vi "FT10_Fornax Read.vi"(8 "error in (no error)":errorcluster, 10 "Timeout":dbl, 11 "TCP Network Connection in":refnum<k5>) -> (0 "error out":errorcluster, 2 "JSON Message":string[](array[string]), 3 "TCP Network Connection out":refnum<k5>)   [LabVIEW 2015]
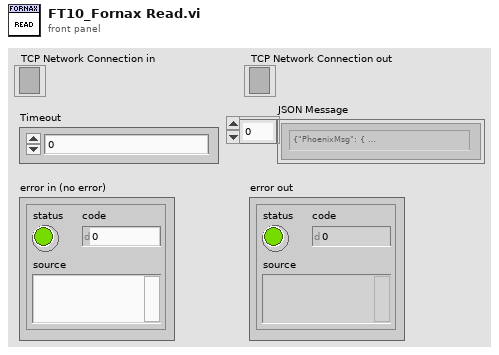
[diagram p1: front panel]
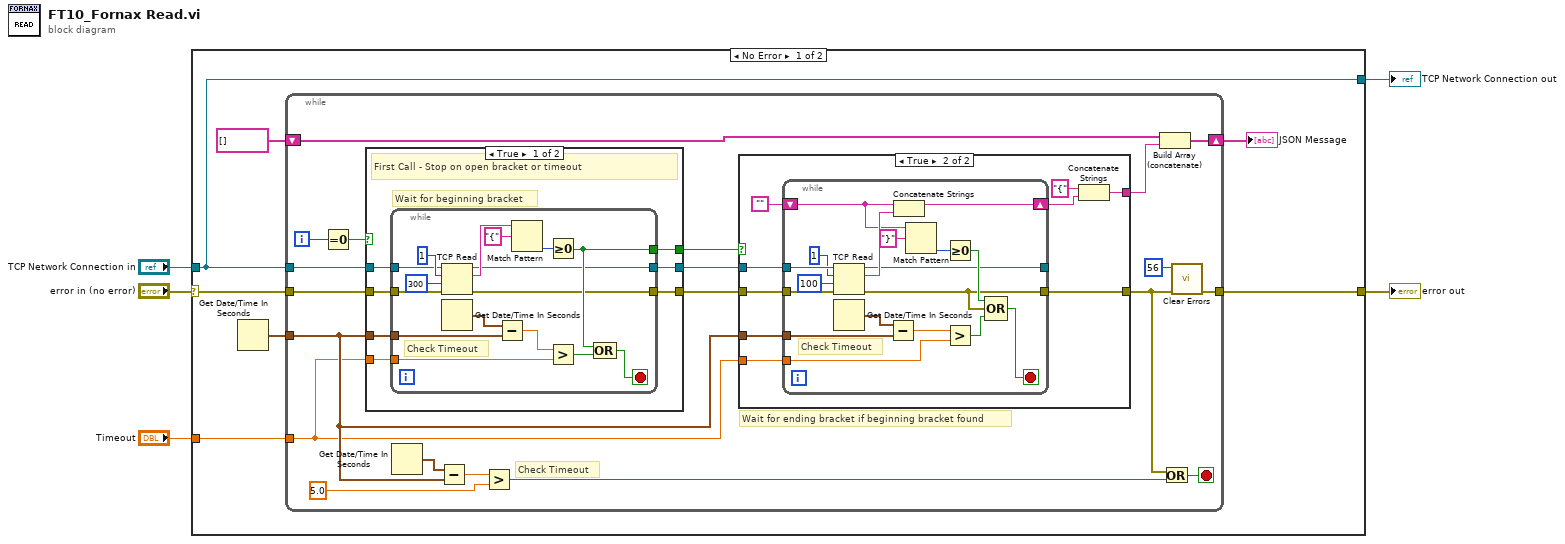
[diagram p0: block diagram]
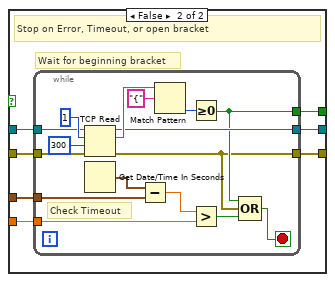
[diagram p2: hidden frame]
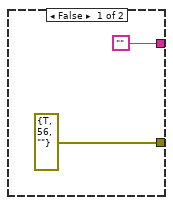
[diagram p3: hidden frame]
diagram:
  n1 = case shown="No Error" "error in (no error)" {
    selector: "error in (no error)" -> [w12 w109]
    tunnel: [w10 w109] -> w2
    tunnel: "TCP Network Connection in" -> [w9 w108]
    tunnel: [w9 w108] -> w4
    tunnel: "Timeout" -> [w8 _]
    frame No Error {
      n2 = Get Date/Time In Seconds() -> (seconds since 1Jan1904=w11:timestamp)
      n3 = while {
        tunnel: w12 -> [w22]
        tunnel: w11 -> [w25]
        tunnel: [w24] -> w10
        tunnel: w8 -> [w20]
        tunnel: w9 -> [w31]
        shift-right: [w17] -> w7
        shift-left: string[] [] ("appended array") -> [w16]
        i -> [w15]
        stop <- w27 stop-if-true
        # "Check Timeout"
        # "Wait for ending bracket if beginning bracket found"
        n4 = Equal To 0?(x=w15) -> (x = 0?=w14:bool)
        n5 = case shown="True" w14 {
          tunnel: [w39 w62] -> w32
          tunnel: w31 -> [w38 w61]
          tunnel: [w37 w60] -> w30
          tunnel: w25 -> [w36 w59]
          tunnel: w22 -> [w35 w58]
          tunnel: w20 -> [w34 w57]
          tunnel: [w33 w56] -> w19
          frame True {
            # "Wait for beginning bracket"
            # "First Call - Stop on open bracket or timeout"
            n6 = while {
              tunnel: w35 -> [w53]
              tunnel: w38 -> [w52]
              tunnel: [w44] -> w39
              tunnel: w36 -> [w48]
              tunnel: [w45] -> w37
              tunnel: w34 -> [w41]
              tunnel: [w40] -> w33
              stop <- w43 stop-if-true
              # "Check Timeout"
              n7 = TCP Read(connection ID=w52, bytes to read=1, error in (no error)=w53, 9:300) -> (connection ID out=w40:refnum<k5>, data out=w47:string, error out=w44:errorcluster)  [unwired: 1 in]
              n8 = Get Date/Time In Seconds() -> (seconds since 1Jan1904=w49:timestamp)
              n9 = Subtract(x=w49, y=w48) -> (x-y=w46:dbl)
              n10 = Match Pattern(string=w47, regular expression="{") -> (offset past match=w50:i32)  [unwired: 1 in, 3 out]
              n11 = Greater Or Equal To 0?(x=w50) -> (x >= 0?=w45:bool)
              n12 = Greater?(x=w46, y=w41) -> (0:w42:bool)
              n13 = Compound Arithmetic op=OR(w45, w42) -> (w43:bool)
            }
          }
          frame False {
            # "Wait for beginning bracket"
            # "Stop on Error, Timeout, or open bracket"
            n14 = while {
              tunnel: w58 -> [w76]
              tunnel: w61 -> [w75]
              tunnel: [w63] -> w62
              tunnel: w59 -> [w71]
              tunnel: [w64] -> w60
              tunnel: w57 -> [w66]
              tunnel: [w65] -> w56
              stop <- w68 stop-if-true
              # "Check Timeout"
              n15 = TCP Read(connection ID=w75, bytes to read=1, error in (no error)=w76, 9:300) -> (connection ID out=w65:refnum<k5>, data out=w70:string, error out=w63:errorcluster)  [unwired: 1 in]
              n16 = Get Date/Time In Seconds() -> (seconds since 1Jan1904=w72:timestamp)
              n17 = Subtract(x=w72, y=w71) -> (x-y=w69:dbl)
              n18 = Match Pattern(string=w70, regular expression="{") -> (offset past match=w73:i32)  [unwired: 1 in, 3 out]
              n19 = Greater Or Equal To 0?(x=w73) -> (x >= 0?=w64:bool)
              n20 = Greater?(x=w69, y=w66) -> (0:w67:bool)
              n21 = Compound Arithmetic op=OR(w64, w63, w67) -> (w68:bool)
            }
          }
        }
        n22 = Get Date/Time In Seconds() -> (seconds since 1Jan1904=w26:timestamp)
        n23 = Subtract(x=w26, y=w25) -> (x-y=w29:dbl)
        n24 = Greater?(x=w29, y=5.0 ("Timeout")) -> (0:w28:bool)
        n25 = case shown="True" w30 {
          tunnel: [errorcluster {"status"=TRUE, "code"=56, "source"=""} ("error out") w89] -> w21
          tunnel: w32 -> [_ w85]
          tunnel: w20 -> [_ w88]
          tunnel: w25 -> [_ w86]
          tunnel: w19 -> [_ w82]
          tunnel: ["" w81] -> w18
          frame False {
          }
          frame True {
            n26 = while {
              tunnel: w85 -> [w107]
              tunnel: [w93] -> w89
              tunnel: w86 -> [w96]
              tunnel: w88 -> [w103]
              shift-right: [w99] -> w83
              shift-left: "" -> [w92]
              tunnel: w82 -> [w106]
              tunnel: [w90] -> _
              stop <- w101 stop-if-true
              # "Check Timeout"
              n27 = TCP Read(connection ID=w106, bytes to read=1, error in (no error)=w107, 9:100 ("timeout ms (25000)")) -> (connection ID out=w90:refnum<k5>, data out=w100:string, error out=w93:errorcluster)  [unwired: 1 in]
              n28 = Get Date/Time In Seconds() -> (seconds since 1Jan1904=w95:timestamp)
              n29 = Subtract(x=w95, y=w96) -> (x-y=w104:dbl)
              n30 = Concatenate Strings(w92, w100) -> (w99:string)
              n31 = Match Pattern(string=w92, regular expression="}") -> (offset past match=w105:i32)  [unwired: 1 in, 3 out]
              n32 = Greater Or Equal To 0?(x=w105) -> (x >= 0?=w94:bool)
              n33 = Greater?(x=w104, y=w103) -> (0:w102:bool)
              n34 = Compound Arithmetic op=OR(w94, w93, w102) -> (w101:bool)
            }
            n35 = Concatenate Strings("{" ("string"), w83) -> (w81:string)
          }
        }
        n36 = Build Array (concatenate)(w16, w18) -> (w17:string[])
        n37 = Or(x=w21, y=w28) -> (x .or. y?=w27:bool)
        n38 = call <vilib>:"Clear Errors.vi"("error in (no error)"=w21, "specific error code to clear (0: all)"=56) -> ("error out"=w24:errorcluster)  [unwired: 4 in, 1 out]
      }
      "JSON Message" <- w7
    }
    frame Error {
    }
  }
  "error out" <- w2
  "TCP Network Connection out" <- w4
